vi "Create Test Method Dialog.vi"(8 "Error In":errorcluster, 11 "Class Ref":refnum<vi>) -> (0 "Error Out":errorcluster, 3 "Cancelled?":bool)   [LabVIEW 2013, in "Scripter.lvlib"]
uses:
  Scripter.lvlib
  _td Dialog Data.ctl
panel:
  in  "_btn Cancel":bool
  in  "_btn OK":bool
  in  "Templates List":u16(ring) items=["test template standart"]
  in  "Use Template?":bool
  out "Log Message":string
  in  "New Test Method Name":string
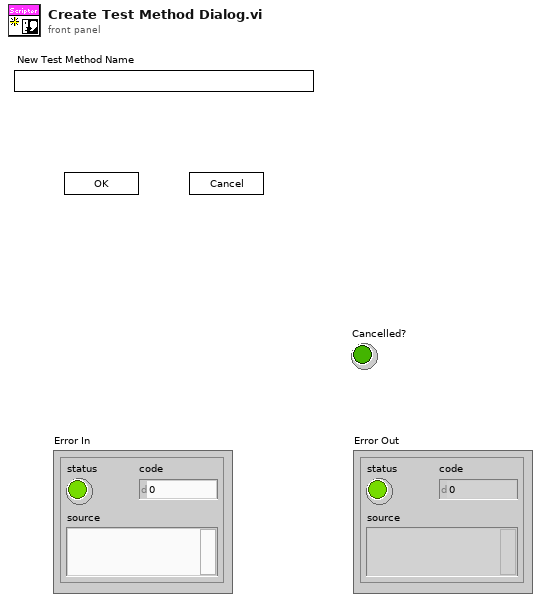
[diagram p1: front panel]
types:
  T1 = enum32{"Invalid", "Standard", "Closed", "Hidden", "Minimized", "Maximized"}
  T2 = enum32{"invalid app kind", "Development System", "Run Time System", "Student Edition", "Embedded LabVIEW", "Evaluation", "Custom"}
  T3 = typedef "Scripter.lvlib/_td Dialog Data.ctl" = cluster{"Core":cluster{"Current VI Reference":refnum<vi>, "Close Panel on Exit?":bool}, "Class Ref":refnum<vi>, "Class Folder Path":path, "Method Name":string, "Methods List":string[], "Templates Folder Path":path, "Template VIs":path[], "Template VIs List":string[], "Use Template?":bool, "Cancelled":bool, "Log Msg":string, "Validation Status":bool, "New Method Path":path, "Class Path":path, "VI Ref":refnum<vi>, "Default Template":path, "Method Idx":i32}
  T4 = enum8{"Enabled", "Disabled", "Disabled and Grayed Out"}
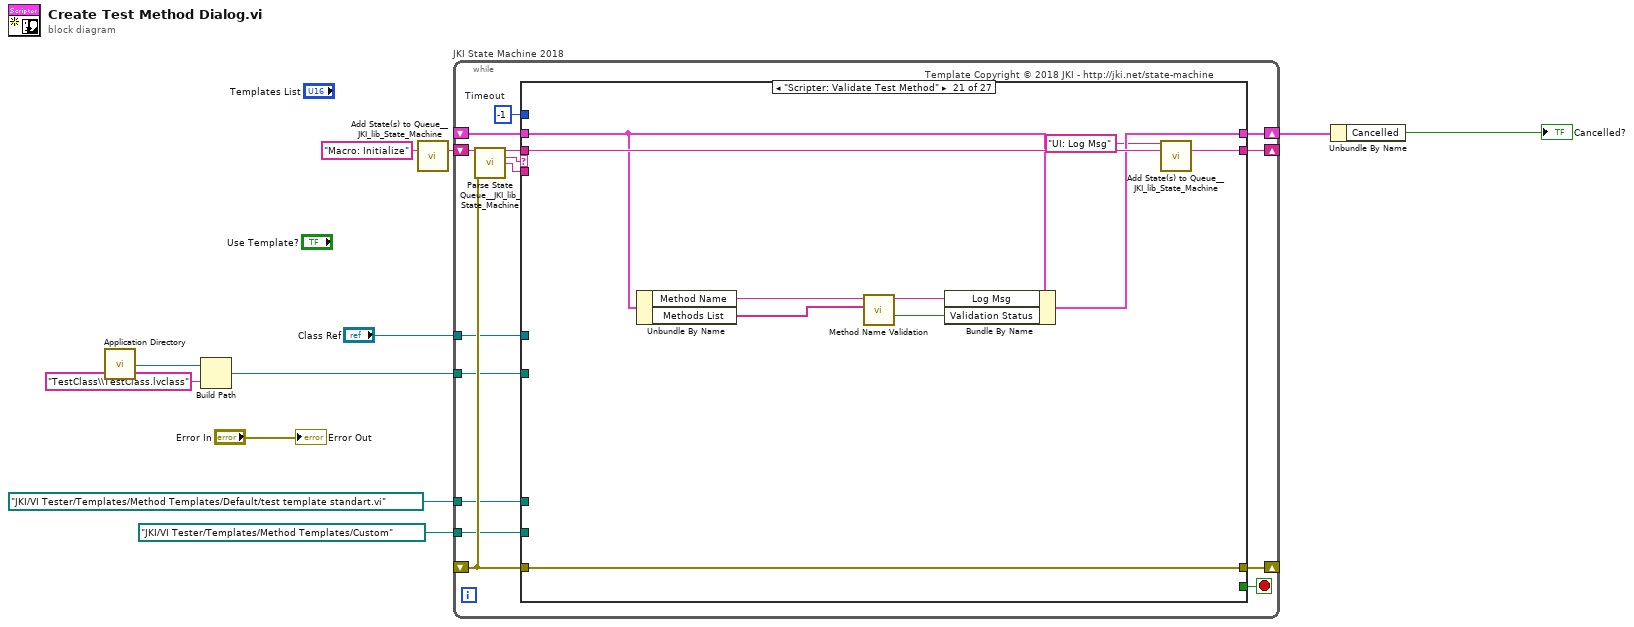
[diagram p0: block diagram]
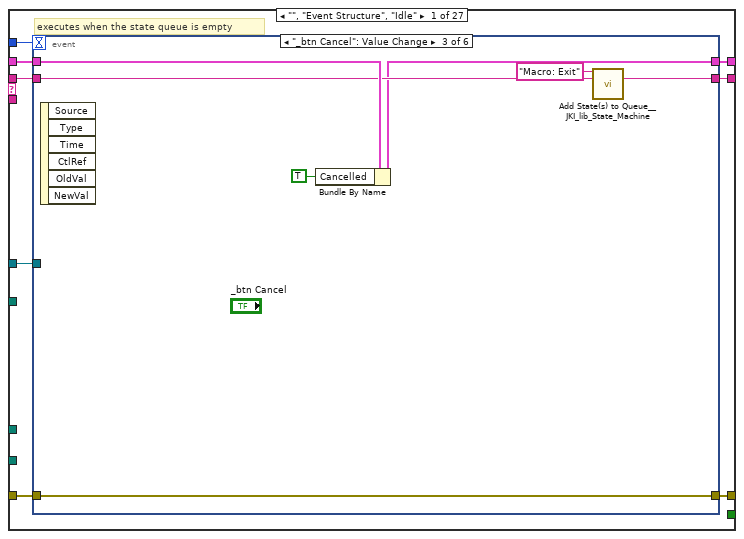
[diagram p2: hidden frame]
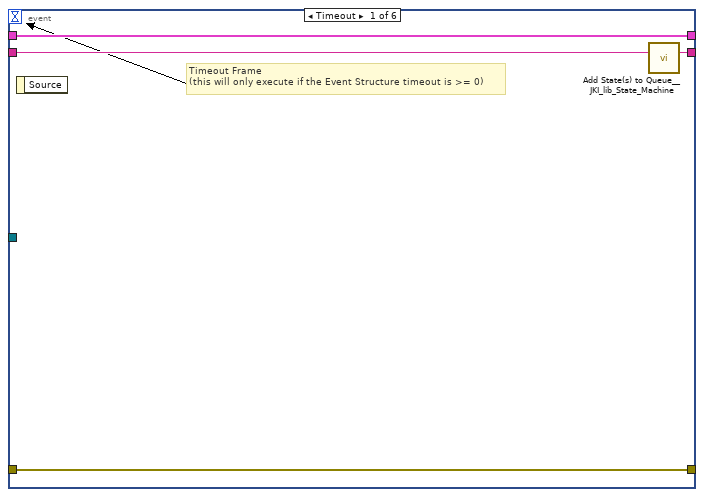
[diagram p3: hidden frame]
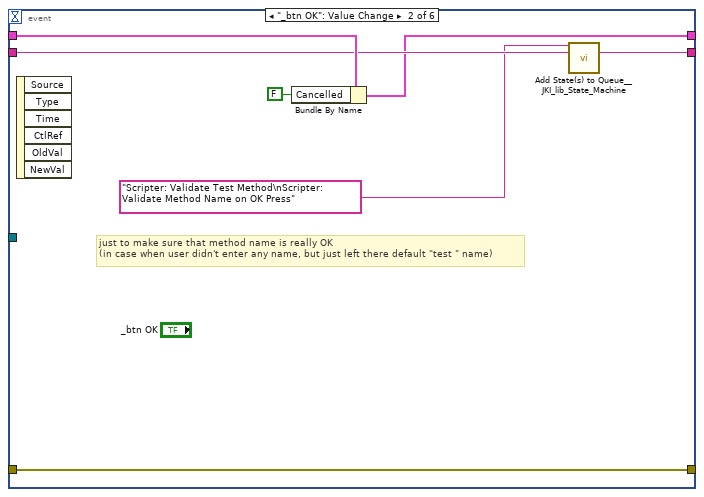
[diagram p4: hidden frame]
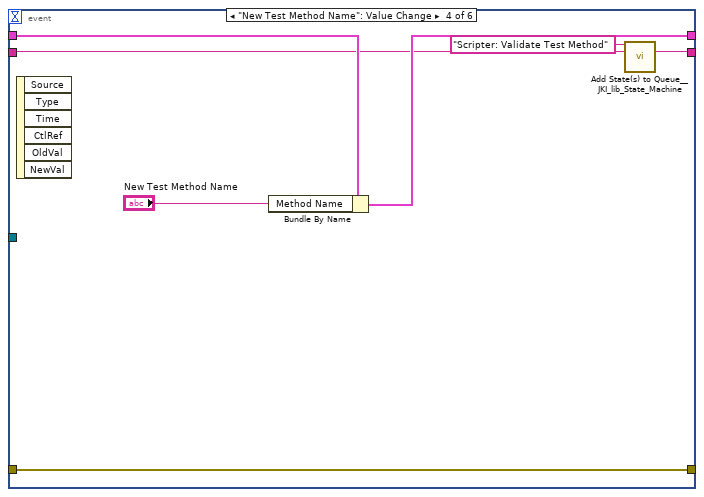
[diagram p5: hidden frame]
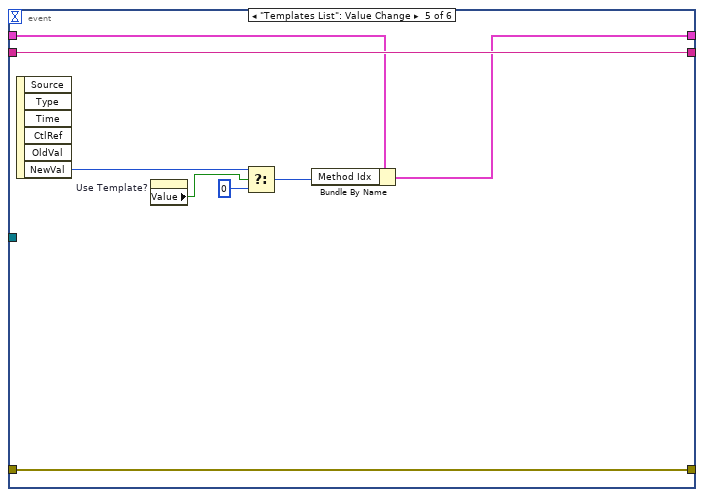
[diagram p6: hidden frame]
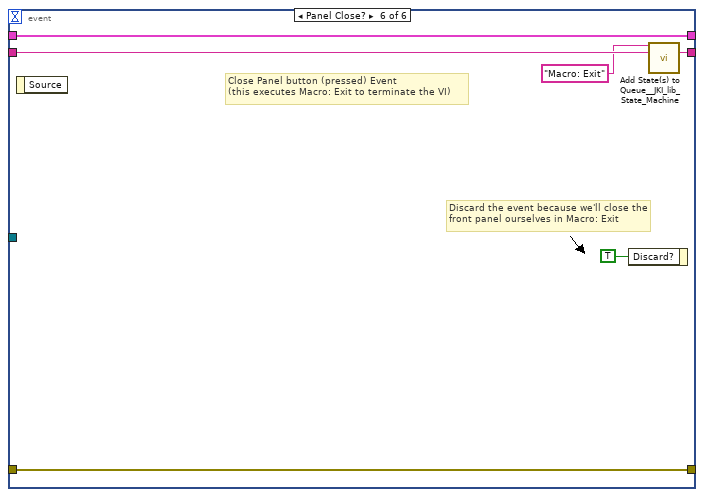
[diagram p7: hidden frame]
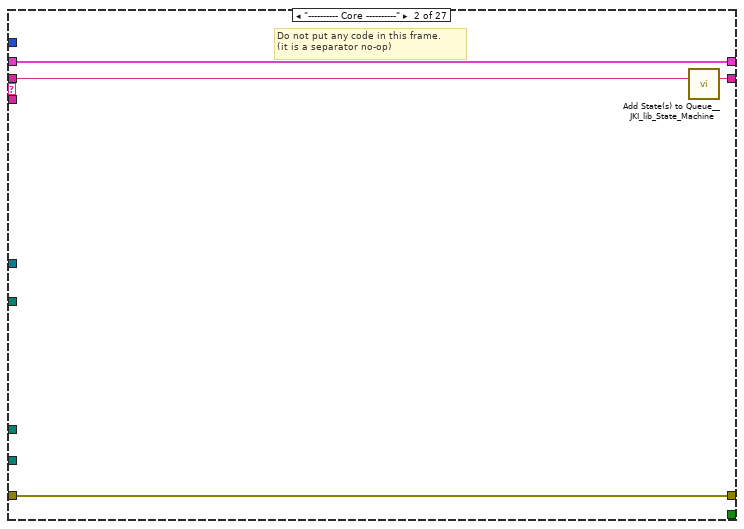
[diagram p8: hidden frame]
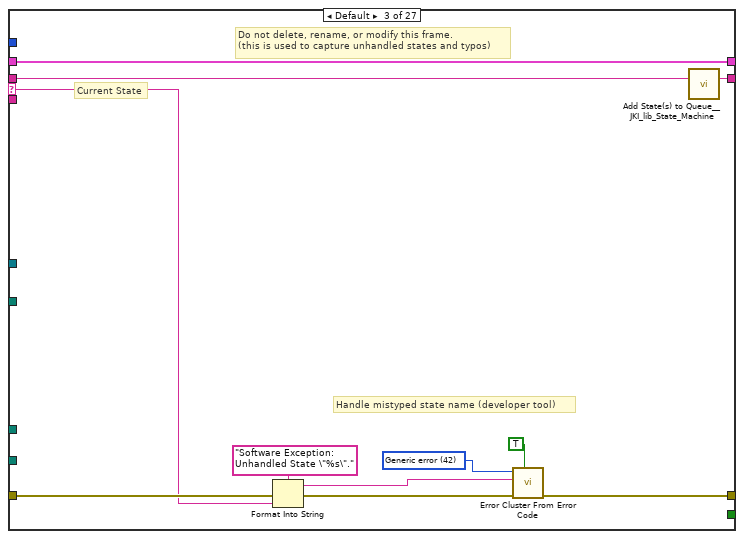
[diagram p9: hidden frame]
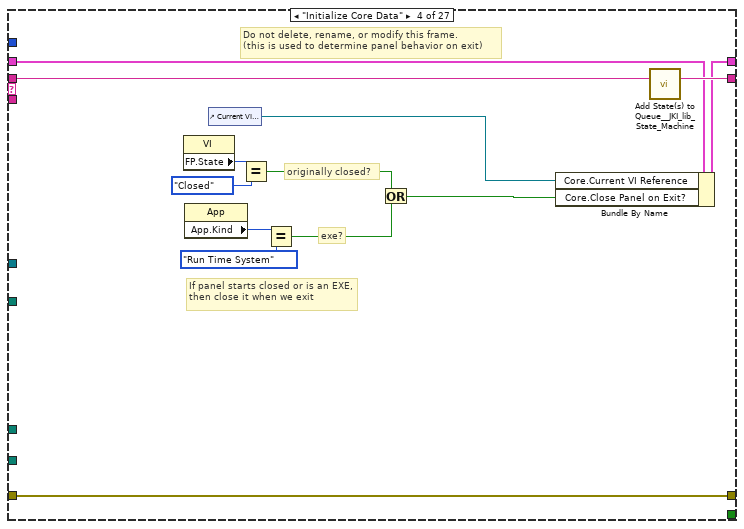
[diagram p10: hidden frame]
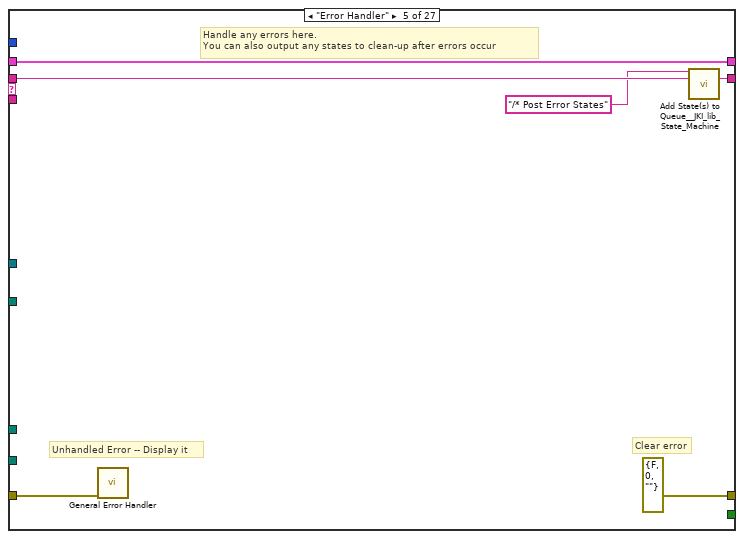
[diagram p11: hidden frame]
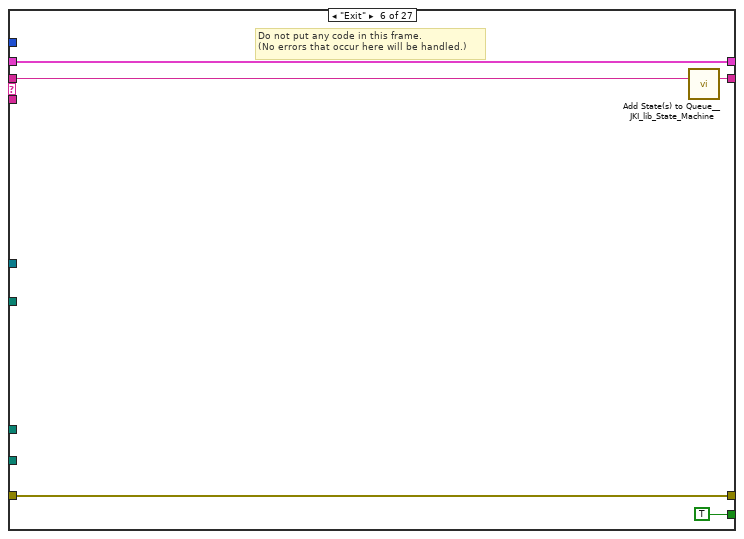
[diagram p12: hidden frame]
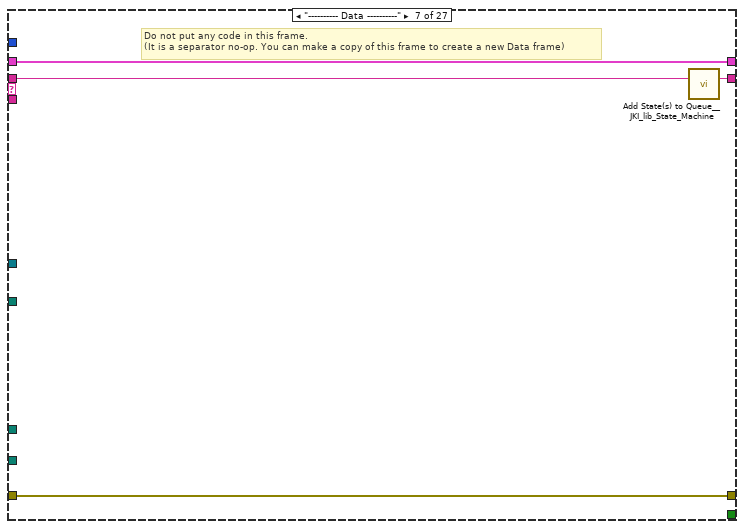
[diagram p13: hidden frame]
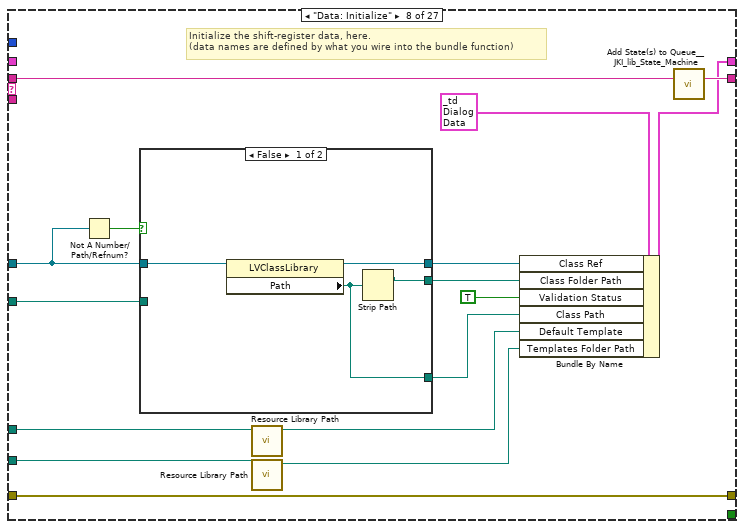
[diagram p14: hidden frame]
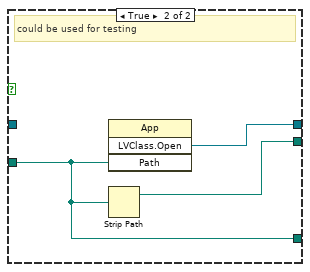
[diagram p15: hidden frame]
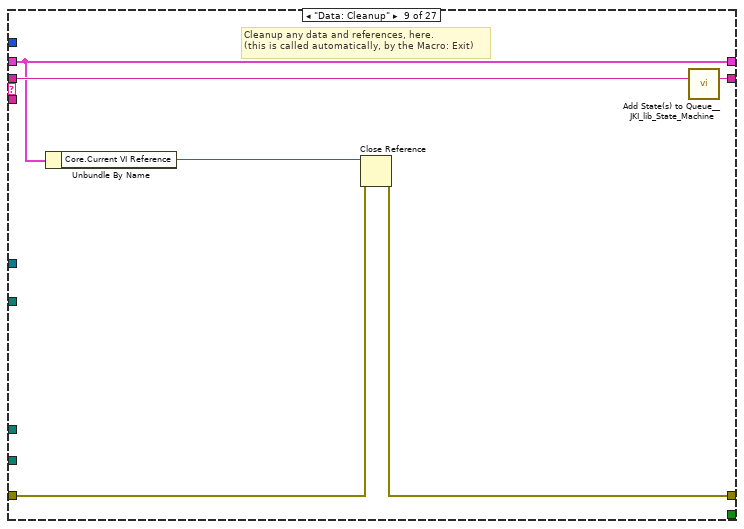
[diagram p16: hidden frame]
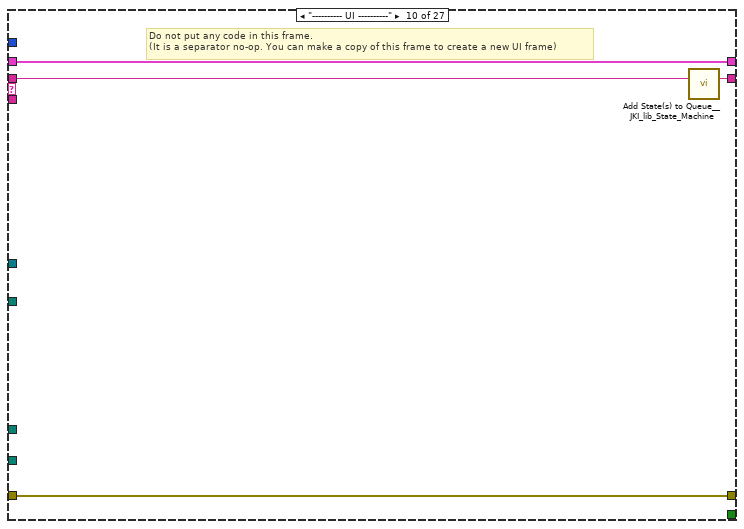
[diagram p17: hidden frame]
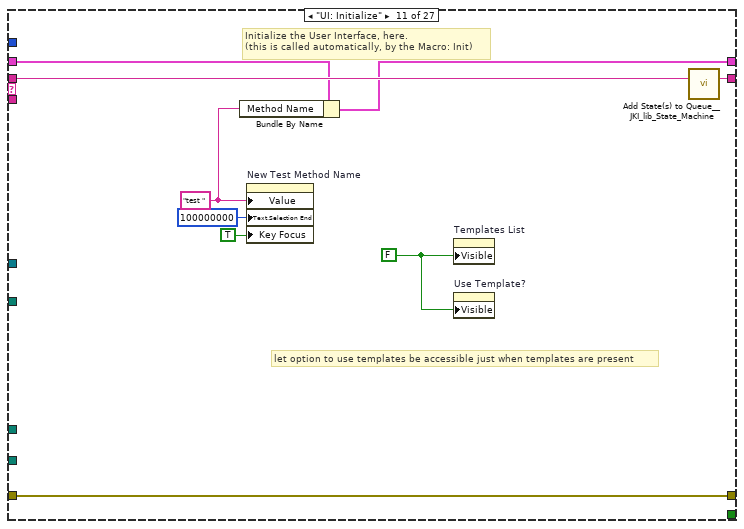
[diagram p18: hidden frame]
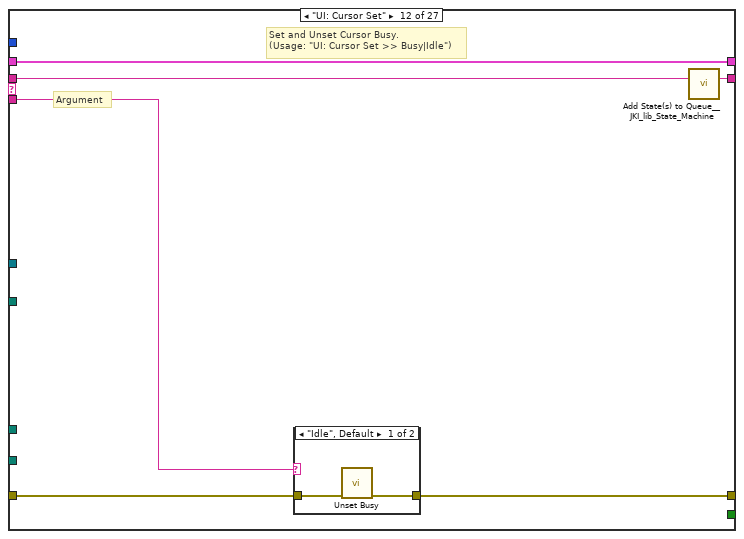
[diagram p19: hidden frame]
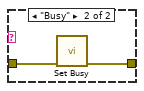
[diagram p20: hidden frame]
diagram:
  n1 = call <vilib>:"Application Directory.vi"() -> ("Application Directory"=w6:path)
  n2 = Build Path(base path=w6, name or relative path="TestClass\\TestClass.lvclass") -> (appended path=w4:path)
  n3 = call <vilib>:"Add State(s) to Queue__JKI_lib_State_Machine.vi"("State(s) in (\"\")"="Macro: Initialize") -> ("States Out"=w11:string)  [unwired: 14 in]
  n4 = while "JKI State Machine 2018" {
    shift-right: [w19] -> w8
    shift-left: _ -> [w18]
    shift-right: [w22] -> _
    shift-left: _ -> [w16]
    shift-right: [w21] -> _
    shift-left: w11 -> [w23]
    tunnel: "Class Ref" -> [w15]
    tunnel: w4 -> [w14]
    tunnel: path "JKI/VI Tester/Templates/Method Templates/Default/test template standart.vi" ("Relative Path") -> [w13]
    tunnel: path "JKI/VI Tester/Templates/Method Templates/Custom" ("Relative Path") -> [w12]
    stop <- w20 stop-if-true
    w17 = -1  # Timeout
    # "Template Copyright © 2018 JKI - http://jki.net/state-machine"
    n5 = call <vilib>:"Parse State Queue__JKI_lib_State_Machine.vi"("State Queue"=w23, "Error In (no error)"=w16) -> ("Remaining States"=w25:string, "Current State"=w26:string, "Arguments"=w24:string)  [unwired: 11 in]
    n6 = case shown="\"Scripter: Validate Test Method\"" w26 {
      selector: w26 -> [_ _ w78 _ _ _ _ _ _ _ _ _ _ _ _ _ _ _ _ _ _ _ _ _ _ _ _]
      tunnel: w25 -> [w34 w77 w82 w101 w107 w112 w116 w132 w145 w149 w158 w164 w175 w249 w256 w262 w267 w272 w282 w286 w296 w304 w314 w330 w340 w352 w363]
      tunnel: w24 -> [_ _ _ _ _ _ _ _ _ _ _ w159 w169 _ _ _ _ _ _ _ _ _ _ _ _ _ _]
      tunnel: w18 -> [w32 w74 w80 w94 w104 w110 w113 _ w140 w146 w156 w162 w171 w246 w253 w259 w264 w269 w279 w283 w293 w301 w311 w324 w337 w350 w361]
      tunnel: [w31 w75 w84 w98 errorcluster {"status"=FALSE, "code"=0, "source"=""} ("error out") w109 w114 w130 w141 w147 w155 w160 w172 w247 w254 w260 w265 w270 w280 w284 w294 w302 w312 w328 w338 w344 w357] -> w22
      tunnel: w16 -> [w30 w75 w83 w98 w103 w109 w114 w130 w142 w147 w155 w161 w173 w247 w254 w260 w265 w270 w280 w284 w294 w302 w312 w328 w338 w345 w358]
      tunnel: [w33 w76 w81 w100 w106 w111 w115 w131 w144 w148 w157 w163 w174 w248 w255 w261 w266 w271 w281 w285 w295 w303 w313 w329 w339 w351 w362] -> w21
      tunnel: [_ _ _ _ _ TRUE _ _ _ _ _ _ _ _ _ _ _ _ _ _ _ _ _ _ _ _ _] -> w20
      tunnel: [w29 w74 w80 w99 w104 w110 w113 w128 w140 w146 w151 w162 w171 w246 w253 w259 w264 w269 w279 w283 w292 w301 w306 w327 w332 w343 w361] -> w19
      tunnel: w17 -> [w28 _ _ _ _ _ _ _ _ _ _ _ _ _ _ _ _ _ _ _ _ _ _ _ _ _ _]
      tunnel: w15 -> [w27 _ _ _ _ _ _ w126 _ _ _ _ _ _ _ _ _ _ _ _ _ _ _ _ _ _ _]
      tunnel: w14 -> [_ _ _ _ _ _ _ w124 _ _ _ _ _ _ _ _ _ _ _ _ _ _ _ _ _ _ _]
      tunnel: w13 -> [_ _ _ _ _ _ _ w119 _ _ _ _ _ _ _ _ _ _ _ _ _ _ _ _ _ _ _]
      tunnel: w12 -> [_ _ _ _ _ _ _ w118 _ _ _ _ _ _ _ _ _ _ _ _ _ _ _ _ _ _ _]
      frame "", "Event Structure", "Idle" {
        # "executes when the state queue is empty"
        n7 = event shown="[2] \"_btn Cancel\": Value Change" {
          selector: _ -> [_ _ _ _ _ _]
          dyn-events: _ -> [_ _ _ _ _ _]
          timeout: w28 -> [_ _ _ _ _ _]
          tunnel: w34 -> [w38 w42 w49 w54 w67 w73]
          tunnel: [w37 w43 w50 w55 w67 w72] -> w33
          tunnel: w32 -> [w35 w44 w51 w58 w65 w70]
          tunnel: [w36 w45 w52 w59 w66 w71] -> w31
          tunnel: w30 -> [w36 w45 w52 w59 w66 w71]
          tunnel: [w35 w40 w47 w57 w64 w70] -> w29
          tunnel: w27 -> [_ _ _ _ _ _]
          event Timeout {
            # "Timeout Frame\n(this will only execute if the Event Structure timeout is >= 0)"
            n8 = event-data() -> ()  [unwired: 1 in, 1 out]
            n9 = call <vilib>:"Add State(s) to Queue__JKI_lib_State_Machine.vi"("State(s) in (\"\")"=w38) -> ("States Out"=w37:string)  [unwired: 14 in]
          }
          event "_btn OK": Value Change {
            # "just to make sure that method name is really OK\n(in case when user didn't enter any name, but just left there default \"test \" name)"
            n10 = event-data() -> ()  [unwired: 1 in, 6 out]
            n11 = Bundle By Name(cluster=w44, "Cancelled"=FALSE) -> (w40:T3)
            n12 = call <vilib>:"Add State(s) to Queue__JKI_lib_State_Machine.vi"("State(s) in Front (\"\")"="Scripter: Validate Test Method\nScripter: Validate Method Name on OK Press" ("State(s) in Front (\"\")"), "State(s) in (\"\")"=w42) -> ("States Out"=w43:string)  [unwired: 13 in]
          }
          event "_btn Cancel": Value Change {
            n13 = event-data() -> ()  [unwired: 1 in, 6 out]
            n14 = Bundle By Name(cluster=w51, "Cancelled"=TRUE) -> (w47:T3)
            n15 = call <vilib>:"Add State(s) to Queue__JKI_lib_State_Machine.vi"("State(s) in Front (\"\")"="Macro: Exit" ("State(s) in Front (\"\")"), "State(s) in (\"\")"=w49) -> ("States Out"=w50:string)  [unwired: 13 in]
          }
          event "New Test Method Name": Value Change {
            n16 = event-data() -> ()  [unwired: 1 in, 6 out]
            n17 = Bundle By Name(cluster=w58, "Method Name"="New Test Method Name") -> (w57:T3)
            n18 = call <vilib>:"Add State(s) to Queue__JKI_lib_State_Machine.vi"("State(s) in Front (\"\")"="Scripter: Validate Test Method" ("State(s) in Front (\"\")"), "State(s) in (\"\")"=w54) -> ("States Out"=w55:string)  [unwired: 13 in]
          }
          event "Templates List": Value Change {
            n19 = event-data() -> ("NewVal"=w62:u16)  [unwired: 1 in, 5 out]
            n20 = property on="Use Template?" class="Bool (strict)"() -> ("Value"=w63:bool)  [unwired: 2 in, 2 out]
            n21 = Select(t=w62, s=w63, f=u16 0) -> (s? t:f=w61:u16)
            n22 = Bundle By Name(cluster=w65, "Method Idx"=w61) -> (w64:T3)
          }
          event Panel Close? {
            # "Discard the event because we'll close the front panel ourselves in Macro: Exit"
            # "Close Panel button (pressed) Event\n(this executes Macro: Exit to terminate the VI)"
            n23 = event-data() -> ()  [unwired: 1 in, 1 out]
            n24 = event-data("Discard?"=TRUE) -> ()  [unwired: 1 in, 1 out]
            n25 = call <vilib>:"Add State(s) to Queue__JKI_lib_State_Machine.vi"("State(s) in Front (\"\")"="Macro: Exit", "State(s) in (\"\")"=w73) -> ("States Out"=w72:string)  [unwired: 13 in]
          }
        }
      }
      frame "---------- Core ----------" {
        # "Do not put any code in this frame.\n(it is a separator no-op)"
        n26 = call <vilib>:"Add State(s) to Queue__JKI_lib_State_Machine.vi"("State(s) in (\"\")"=w77) -> ("States Out"=w76:string)  [unwired: 14 in]
      }
      frame Default {
        w87 = 42 items=["No error", "Argument error", "Memory is full", "Out of zone", "End of file", "File already open", "Generic file I/O error", "File not found", "File permission error", "Disk is full", "Duplicate path", "Too many files open", "System feature not enabled", "Resource file not found", "Cannot add resource", "Resource not found", "Image not found", "Image memory error", "Pen does not exist", "Config type invalid", "Config token not found", "Config parse error", "Config memory error", "Bad external code format", "Bad external code offset", "External code not present", "Null window", "Destroy window error", "Null menu", "Print aborted", "Bad print record", "Print driver error", "Windows error during printing", "Memory error during printing", "Print dialog error", "Generic print error", "Invalid device refnum", "Device not found", "Device parameter error", "Device unit error", "Cannot open device", "Device call aborted", "Generic error", "Cancelled by user", "Object ID too low", "Object ID too high", "Object not in heap", "Unknown heap", "Unknown object (invalid DefProc)", "Unknown object (DefProc not in table)", "Message out of range", "Invalid (null) method", "Unknown message", "Manager call not supported", "Bad address", "Network operation in progress", "Network operation timed out", "Connection is busy", "Network attribute not supported", "Network error", "Address in use", "System out of memory", "Connection aborted", "Connection refused", "Not connected", "Already connected", "Connection closed", "Initialization error (interapplication manager)", "Bad occurrence", "Wait on unbound occurrence handler", "Occurrence queue overflow", "Datalog type conflict", "Unused", "Unrecognized type (interapplication manager)", "Memory corrupt", "Failed to make temporary DLL", "Old CIN version", "Drag socket not found", "Failed to load drop-object", "Failed to register OLE object", "Failed to release OLE object", "Format specifier type mismatch", "Unknown format specifier", "Too few format specifiers", "Too many format specifiers", "Scan failed", "Newer CIN version", "Error converting to variant", "Runtime menu error", "Password tampered", "Variant attribute not found", "Incompatible variant data type", "Event data is not available", "Event Store is not present", "Occurrence is not found", "Event Queue is not created", "Event info is not available", "Refnum passed is NULL", "Error retrieving Class GUID", "Error retrieving CoClass GUID", "Error retrieving TypeLib GUID.", "Bad built application magic bytes.", "Specific driver is different from the specific driver associated with the Logical Name.", "There is no session opened to the class driver.", "Max Error", "MAX - Error with config objects", "MAX - Error loading configuration", "MAX - Group not supported"]
        # "Current State"
        # "Do not delete, rename, or modify this frame.\n(this is used to capture unhandled states and typos)"
        # "Handle mistyped state name (developer tool)"
        n27 = Format Into String(format string="Software Exception: Unhandled State \"%s\"." ("message"), error in=w83, w78) -> (resulting string=w86:string, error out=w85:errorcluster)  [unwired: 1 in]
        n28 = call <vilib>:"Error Cluster From Error Code.vi"("show call chain? (False)"=TRUE, "error in (no error)"=w85, "error message (\"\")"=w86, "error code (0)"=w87) -> ("error out"=w84:errorcluster)  [unwired: 5 in]
        n29 = call <vilib>:"Add State(s) to Queue__JKI_lib_State_Machine.vi"("State(s) in (\"\")"=w82) -> ("States Out"=w81:string)  [unwired: 14 in]
      }
      frame "Initialize Core Data" {
        # "Do not delete, rename, or modify this frame.\n(this is used to determine panel behavior on exit)"
        # "originally closed?"
        # "exe?"
        # "If panel starts closed or is an EXE, then close it when we exit"
        n30 = property class="VI"() -> ("FP.State"=w91:T1)  [unwired: 2 in, 2 out]
        n31 = property class="App"() -> ("App.Kind"=w97:T2)  [unwired: 2 in, 2 out]
        n32 = control-ref of="Current VI Reference"() -> (w92:refnum<vi>)
        n33 = Equal?(x=w91, y=T1."Closed" ("Front Panel Window:State")) -> (x = y?=w89:bool)
        n34 = Equal?(x=w97, y=T2."Run Time System" ("Application:Kind")) -> (x = y?=w95:bool)
        n35 = Or(x=w89, y=w95) -> (x .or. y?=w93:bool)
        n36 = Bundle By Name(cluster=w94, "Core.Current VI Reference"=w92, "Core.Close Panel on Exit?"=w93) -> (w99:T3)
        n37 = call <vilib>:"Add State(s) to Queue__JKI_lib_State_Machine.vi"("State(s) in (\"\")"=w101) -> ("States Out"=w100:string)  [unwired: 14 in]
      }
      frame "Error Handler" {
        # "Unhandled Error -- Display it"
        # "Handle any errors here.\nYou can also output any states to clean-up after errors occur"
        # "Clear error"
        n38 = call <vilib>:"General Error Handler.vi"("error in (no error)"=w103) -> ()  [unwired: 10 in, 5 out]
        n39 = call <vilib>:"Add State(s) to Queue__JKI_lib_State_Machine.vi"("State(s) in Front (\"\")"="/* Post Error States", "State(s) in (\"\")"=w107) -> ("States Out"=w106:string)  [unwired: 13 in]
      }
      frame "Exit" {
        # "Do not put any code in this frame.\n(No errors that occur here will be handled.)"
        n40 = call <vilib>:"Add State(s) to Queue__JKI_lib_State_Machine.vi"("State(s) in (\"\")"=w112) -> ("States Out"=w111:string)  [unwired: 14 in]
      }
      frame "---------- Data ----------" {
        # "Do not put any code in this frame.\n(It is a separator no-op. You can make a copy of this frame to create a new Data frame)"
        n41 = call <vilib>:"Add State(s) to Queue__JKI_lib_State_Machine.vi"("State(s) in (\"\")"=w116) -> ("States Out"=w115:string)  [unwired: 14 in]
      }
      frame "Data: Initialize" {
        # "Initialize the shift-register data, here.\n(data names are defined by what you wire into the bundle function)"
        n42 = Not A Number/Path/Refnum?(number/path/refnum=w126) -> (NaN/Path/Refnum?=w127:bool)
        n43 = case shown="False" w127 {
          tunnel: w126 -> [w136 _]
          tunnel: [w135 w139] -> w125
          tunnel: w124 -> [_ w137]
          tunnel: [w134 w138] -> w123
          tunnel: [w133 w137] -> w121
          frame False {
            n44 = property class="LVClassLibrary"(reference=w136) -> (reference out=w135:refnum<vi>, "Path"=w133:path)  [unwired: 1 in, 1 out]
            n45 = Strip Path(path=w133) -> (stripped path=w134:path)  [unwired: 1 out]
          }
          frame True {
            # "could be used for testing"
            n46 = invoke class="App" method="LVClass.Open"("Path"=w137) -> ("LVClass.Open"=w139:refnum<vi>)  [unwired: 3 in, 3 out]
            n47 = Strip Path(path=w137) -> (stripped path=w138:path)  [unwired: 1 out]
          }
        }
        n48 = call "Resource Library Path.vi"("Relative Path"=w119) -> ("Resource + Relative Path"=w120:path)  [unwired: 10 in]
        n49 = call "Resource Library Path.vi"("Relative Path"=w118) -> ("Resource + Relative Path"=w117:path)  [unwired: 10 in]
        n50 = Bundle By Name(cluster=T3 {"Core"={"Current VI Reference"=refnum, "Close Panel on Exit?"=FALSE}, "Class Ref"=refnum, "Class Folder Path"=path "", "Method Name"="", "Methods List"=[], "Templates Folder Path"=path "", "Template VIs"=[], "Template VIs List"=[], "Use Template?"=FALSE, "Cancelled"=FALSE, "Log Msg"="", "Validation Status"=FALSE, "New Method Path"=path "", "Class Path"=path "", "VI Ref"=refnum, "Default Template"=path "", "Method Idx"=0} ("Dialog Data"), "Class Ref"=w125, "Class Folder Path"=w123, "Validation Status"=TRUE, "Class Path"=w121, "Default Template"=w120, "Templates Folder Path"=w117) -> (w128:T3)
        n51 = call <vilib>:"Add State(s) to Queue__JKI_lib_State_Machine.vi"("State(s) in (\"\")"=w132) -> ("States Out"=w131:string)  [unwired: 14 in]
      }
      frame "Data: Cleanup" {
        # "Cleanup any data and references, here.\n(this is called automatically, by the Macro: Exit)"
        n52 = Unbundle By Name(w140) -> ("Core.Current VI Reference"=w143:refnum<vi>)
        n53 = Close Reference(reference=w143, error in (no error)=w142) -> (error out=w141:errorcluster)
        n54 = call <vilib>:"Add State(s) to Queue__JKI_lib_State_Machine.vi"("State(s) in (\"\")"=w145) -> ("States Out"=w144:string)  [unwired: 14 in]
      }
      frame "---------- UI ----------" {
        # "Do not put any code in this frame.\n(It is a separator no-op. You can make a copy of this frame to create a new UI frame)"
        n55 = call <vilib>:"Add State(s) to Queue__JKI_lib_State_Machine.vi"("State(s) in (\"\")"=w149) -> ("States Out"=w148:string)  [unwired: 14 in]
      }
      frame "UI: Initialize" {
        w150 = "test " ("New Test Method Name")
        w154 = FALSE ("Visible")
        # "let option to use templates be accessible just when templates are present"
        # "Initialize the User Interface, here.\n(this is called automatically, by the Macro: Init)"
        n56 = Bundle By Name(cluster=w156, "Method Name"=w150) -> (w151:T3)
        n57 = property on="New Test Method Name" class="Str"("Value"=w150, "Text.Selection End"=u32 100000000 ("Text.Selection:End"), "Key Focus"=TRUE) -> ()  [unwired: 2 in, 2 out]
        n58 = property on="Templates List" class="Ring (strict)"("Visible"=w154) -> ()  [unwired: 2 in, 2 out]
        n59 = property on="Use Template?" class="Bool (strict)"("Visible"=w154) -> ()  [unwired: 2 in, 2 out]
        n60 = call <vilib>:"Add State(s) to Queue__JKI_lib_State_Machine.vi"("State(s) in (\"\")"=w158) -> ("States Out"=w157:string)  [unwired: 14 in]
      }
      frame "UI: Cursor Set" {
        # "Argument"
        # "Set and Unset Cursor Busy.\n(Usage: \"UI: Cursor Set >> Busy|Idle\")"
        n61 = case shown="\"Idle\", Default" w159 {
          tunnel: w161 -> [w166 w168]
          tunnel: [w165 w167] -> w160
          frame "Idle", Default {
            n62 = call <vilib>:"Unset Busy.vi"("error in (no error)"=w166) -> ("error out"=w165:errorcluster)  [unwired: 10 in]
          }
          frame "Busy" {
            n63 = call <vilib>:"Set Busy.vi"("error in (no error)"=w168) -> ("error out"=w167:errorcluster)  [unwired: 9 in, 1 out]
          }
        }
        n64 = call <vilib>:"Add State(s) to Queue__JKI_lib_State_Machine.vi"("State(s) in (\"\")"=w164) -> ("States Out"=w163:string)  [unwired: 14 in]
      }
      frame "UI: Front Panel State" {
        # "Argument"
        # "Set Front Panel Open or Closed\n(Usage: \"UI: Front Panel State >> Open|Close\")"
        n65 = Unbundle By Name(w171) -> ("Core.Current VI Reference"=w170:refnum<vi>)
        n66 = case shown="\"Open\", \"Standard\", Default" w169 {
          tunnel: w173 -> [w181 w196 w207 w220 w233]
          tunnel: [w183 w197 w209 w222 w235] -> w172
          tunnel: w170 -> [w182 w194 w208 w221 w234]
          frame "Open", "Standard", Default {
            w176 = T1."Standard" ("State")
            n67 = property class="VI"(reference=w182, error in=w181) -> (reference out=w179:refnum<vi>, error out=w180:errorcluster, "FP.State"=w178:T1)
            n68 = Not Equal?(x=w178, y=w176) -> (x != y?=w177:bool)
            n69 = case shown="True" w177 {
              tunnel: [w187 w189] -> w183
              tunnel: w180 -> [w186 w189]
              tunnel: w179 -> [w185 _]
              tunnel: w176 -> [w184 _]
              frame True {
                n70 = invoke class="VI" method="FP.Open"(reference=w185, error in=w186, "Activate"=TRUE, "State"=w184) -> (error out=w187:errorcluster)  [unwired: 1 in, 4 out]
              }
              frame False {
              }
            }
          }
          frame "Close", "Closed" {
            n71 = property class="VI"(reference=w194, error in=w196) -> (reference out=w193:refnum<vi>, error out=w195:errorcluster, "FP.State"=w191:T1)
            n72 = Not Equal?(x=w191, y=T1."Closed" ("Front Panel Window:State")) -> (x != y?=w190:bool)
            n73 = case shown="True" w190 {
              tunnel: [w198 w201] -> w197
              tunnel: w195 -> [w198 w200]
              tunnel: w193 -> [_ w199]
              frame False {
              }
              frame True {
                n74 = invoke class="VI" method="FP.Close"(reference=w199, error in=w200) -> (error out=w201:errorcluster)  [unwired: 1 in, 2 out]
              }
            }
          }
          frame "Hidden", "Hide" {
            w202 = T1."Hidden" ("State")
            n75 = property class="VI"(reference=w208, error in=w207) -> (reference out=w205:refnum<vi>, error out=w206:errorcluster, "FP.State"=w204:T1)
            n76 = Not Equal?(x=w204, y=w202) -> (x != y?=w203:bool)
            n77 = case shown="True" w203 {
              tunnel: [w213 w214] -> w209
              tunnel: w206 -> [w212 w214]
              tunnel: w205 -> [w211 _]
              tunnel: w202 -> [w210 _]
              frame True {
                n78 = invoke class="VI" method="FP.Open"(reference=w211, error in=w212, "State"=w210) -> (error out=w213:errorcluster)  [unwired: 2 in, 4 out]
              }
              frame False {
              }
            }
          }
          frame "Minimize", "Minimized" {
            w215 = T1."Minimized" ("State")
            n79 = property class="VI"(reference=w221, error in=w220) -> (reference out=w218:refnum<vi>, error out=w219:errorcluster, "FP.State"=w217:T1)
            n80 = Not Equal?(x=w217, y=w215) -> (x != y?=w216:bool)
            n81 = case shown="True" w216 {
              tunnel: [w226 w227] -> w222
              tunnel: w219 -> [w225 w227]
              tunnel: w218 -> [w224 _]
              tunnel: w215 -> [w223 _]
              frame True {
                n82 = invoke class="VI" method="FP.Open"(reference=w224, error in=w225, "State"=w223) -> (error out=w226:errorcluster)  [unwired: 2 in, 4 out]
              }
              frame False {
              }
            }
          }
          frame "Maximize", "Maximized" {
            w228 = T1."Maximized" ("State")
            n83 = property class="VI"(reference=w234, error in=w233) -> (reference out=w231:refnum<vi>, error out=w232:errorcluster, "FP.State"=w230:T1)
            n84 = Not Equal?(x=w230, y=w228) -> (x != y?=w229:bool)
            n85 = case shown="True" w229 {
              tunnel: [w239 w240] -> w235
              tunnel: w232 -> [w238 w240]
              tunnel: w231 -> [w237 _]
              tunnel: w228 -> [w236 _]
              frame True {
                n86 = invoke class="VI" method="FP.Open"(reference=w237, error in=w238, "State"=w236) -> (error out=w239:errorcluster)  [unwired: 2 in, 4 out]
              }
              frame False {
              }
            }
          }
        }
        n87 = call <vilib>:"Add State(s) to Queue__JKI_lib_State_Machine.vi"("State(s) in (\"\")"=w175) -> ("States Out"=w174:string)  [unwired: 14 in]
      }
      frame "UI: Log Msg" {
        n88 = Unbundle By Name(w246) -> ("Log Msg"=→"Log Message":string, "Validation Status"=w244:bool)
        n89 = Select(t=T4."Enabled" ("Disabled"), s=w244, f=T4."Disabled and Grayed Out" ("Disabled")) -> (s? t:f=w243:T4)
        n90 = property on="_btn OK" class="Bool"("DisabledEnum"=w243) -> ()  [unwired: 2 in, 2 out]
        n91 = call <vilib>:"Add State(s) to Queue__JKI_lib_State_Machine.vi"("State(s) in (\"\")"=w249) -> ("States Out"=w248:string)  [unwired: 14 in]
      }
      frame "UI: Display Templates List" {
        n92 = Unbundle By Name(w253) -> ("Template VIs"=w251:path[])
        n93 = for {
          tunnel: w251 -> [w258] mode=indexing
          tunnel: [w257] -> w250 mode=indexing
          n94 = call <vilib>:"Get File Extension.vi"("file"=w258) -> ("filename without extension"=w257:string)  [unwired: 7 in, 3 out]
        }
        n95 = property on="Templates List" class="Ring (strict)"("Strings []"=w250, "Value"=0) -> ()  [unwired: 2 in, 2 out]
        n96 = call <vilib>:"Add State(s) to Queue__JKI_lib_State_Machine.vi"("State(s) in (\"\")"=w256) -> ("States Out"=w255:string)  [unwired: 14 in]
      }
      frame "---------- Macro ----------" {
        # "Do not put any code in this frame.\n(It is a separator no-op. You can make a copy of this frame to create a new Macro frame)"
        n97 = call <vilib>:"Add State(s) to Queue__JKI_lib_State_Machine.vi"("State(s) in (\"\")"=w262) -> ("States Out"=w261:string)  [unwired: 14 in]
      }
      frame "Macro: Initialize" {
        w263 = "Data: Initialize\nInitialize Core Data\nUI: Initialize\nUI: Log Msg\nUI: Front Panel State >> Open\nScripter: Get Methods List\nScripter: Get Templates List"  # Data: Initialize Initialize Core Data UI: Initialize UI: Log Msg UI: Front Panel State >> Open Scripter: Get Methods List Scripter: Get Templates List
        # "Initialization Macro\n(This is called once, when the VI starts)"
        n98 = call <vilib>:"Add State(s) to Queue__JKI_lib_State_Machine.vi"("State(s) in Front (\"\")"=w263, "State(s) in (\"\")"=w267) -> ("States Out"=w266:string)  [unwired: 13 in]
      }
      frame "Macro: Add Test Method" {
        n99 = call <vilib>:"Add State(s) to Queue__JKI_lib_State_Machine.vi"("State(s) in Front (\"\")"="Scripter: Prepare Paths\nScripter: Generate VI\nScripter: Add VI to Class\nMacro: Exit" ("State(s) in Front (\"\")"), "State(s) in (\"\")"=w272) -> ("States Out"=w271:string)  [unwired: 13 in]
      }
      frame "Macro: Exit" {
        # "Exit Macro\n(This is called once, when the VI exits)"
        n100 = Unbundle By Name(w279) -> ("Core.Close Panel on Exit?"=w278:bool)
        n101 = Select(t="UI: Front Panel State >> Close", s=w278, f="") -> (s? t:f=w275:string)
        n102 = call <vilib>:"Add State(s) to Queue__JKI_lib_State_Machine.vi"("State(s) in (\"\")"=w275, "State(s) at Back (\"\")"="Data: Cleanup\nExit") -> ("States Out"=w273:string)  [unwired: 13 in]
        n103 = call <vilib>:"Add State(s) to Queue__JKI_lib_State_Machine.vi"("State(s) in Front (\"\")"=w273, "State(s) in (\"\")"=w282) -> ("States Out"=w281:string)  [unwired: 13 in]
      }
      frame "---------- Scripter ----------" {
        # "Template Separator\n(You can make a copy of, or modify, this frame)"
        n104 = call <vilib>:"Add State(s) to Queue__JKI_lib_State_Machine.vi"("State(s) in (\"\")"=w286) -> ("States Out"=w285:string)  [unwired: 14 in]
      }
      frame "Scripter: Validate Test Method" {
        n105 = Unbundle By Name(w293) -> ("Method Name"=w287:string, "Methods List"=w288:string[])
        n106 = call "Method Name Validation.vi"("Methods List in"=w288, "Method Name in"=w287) -> ("Validation Status out"=w289:bool, "Log Message out"=w291:string)  [unwired: 8 in]
        n107 = Bundle By Name(cluster=w293, "Log Msg"=w291, "Validation Status"=w289) -> (w292:T3)
        n108 = call <vilib>:"Add State(s) to Queue__JKI_lib_State_Machine.vi"("State(s) in Front (\"\")"="UI: Log Msg", "State(s) in (\"\")"=w296) -> ("States Out"=w295:string)  [unwired: 13 in]
      }
      frame "Scripter: Validate Method Name on OK Press" {
        # "Template Separator\n(You can make a copy of, or modify, this frame)"
        n109 = Unbundle By Name(w301) -> ("Validation Status"=w300:bool)
        n110 = Select(t="Macro: Add Test Method" ("State(s) in Front (\"\")"), s=w300, f="") -> (s? t:f=w297:string)
        n111 = call <vilib>:"Add State(s) to Queue__JKI_lib_State_Machine.vi"("State(s) in Front (\"\")"=w297, "State(s) in (\"\")"=w304) -> ("States Out"=w303:string)  [unwired: 13 in]
      }
      frame "Scripter: Get Methods List" {
        n112 = Unbundle By Name(w311) -> ("Class Ref"=w310:refnum<vi>)
        n113 = property class="LVClassLibrary"(reference=w310) -> ("Dynamic Member VIs"=w309:refnum<vi>[], "Static Member VIs"=w308:refnum<vi>[])  [unwired: 1 in, 2 out]
        n114 = Build Array (concatenate)(w309, w308) -> (w307:refnum<vi>[])
        n115 = for {
          tunnel: w307 -> [w317] mode=indexing
          tunnel: [w315] -> w305 mode=indexing
          n116 = property class="VI"(reference=w317) -> ("Path"=w316:path)  [unwired: 1 in, 2 out]
          n117 = call <vilib>:"Get File Extension.vi"("file"=w316) -> ("filename without extension"=w315:string)  [unwired: 7 in, 3 out]
        }
        n118 = Bundle By Name(cluster=w311, "Methods List"=w305) -> (w306:T3)
        n119 = call <vilib>:"Add State(s) to Queue__JKI_lib_State_Machine.vi"("State(s) in (\"\")"=w314) -> ("States Out"=w313:string)  [unwired: 14 in]
      }
      frame "Scripter: Get Templates List" {
        n120 = Unbundle By Name(w324) -> ("Default Template"=w321:path, "Templates Folder Path"=w323:path)
        n121 = call <vilib>:"Recursive File List.vi"("pattern"="*.vi", "Folder Path"=w323) -> ("All Files in Dir"=w320:path[])  [unwired: 5 in, 4 out]
        n122 = Build Array (concatenate)(w321, w320) -> (w319:path[])
        n123 = Empty Array?(array=w320) -> (empty?=w326:bool)
        n124 = Not(x=w326) -> (.not. x?=w325:bool)
        n125 = Bundle By Name(cluster=w324, "Template VIs"=w319) -> (w327:T3)
        n126 = property on="Templates List" class="Ring (strict)"("Visible"=w325) -> ()  [unwired: 2 in, 2 out]
        n127 = property on="Use Template?" class="Bool (strict)"("Visible"=w325) -> ()  [unwired: 2 in, 2 out]
        n128 = call <vilib>:"Add State(s) to Queue__JKI_lib_State_Machine.vi"("State(s) in Front (\"\")"="UI: Display Templates List" ("State(s) in Front (\"\")"), "State(s) in (\"\")"=w330) -> ("States Out"=w329:string)  [unwired: 13 in]
      }
      frame "Scripter: Prepare Paths" {
        n129 = Unbundle By Name(w337) -> ("Class Folder Path"=w333:path, "Method Name"=w336:string)
        n130 = Format Into String(format string="%s.vi", w336) -> (resulting string=w334:string)  [unwired: 2 in, 1 out]
        n131 = Build Path(base path=w333, name or relative path=w334) -> (appended path=w331:path)
        n132 = Bundle By Name(cluster=w337, "New Method Path"=w331) -> (w332:T3)
        n133 = call <vilib>:"Add State(s) to Queue__JKI_lib_State_Machine.vi"("State(s) in (\"\")"=w340) -> ("States Out"=w339:string)  [unwired: 14 in]
      }
      frame "Scripter: Generate VI" {
        # "Template Separator\n(You can make a copy of, or modify, this frame)"
        n134 = Unbundle By Name(w350) -> ("Template VIs"=w349:path[], "Method Idx"=w341:i32, "Class Path"=w347:path, "New Method Path"=w346:path)
        n135 = Index Array(array=w349, index=w341) -> (element=w348:path)
        n136 = call "Replace Class Inputs.vi"("Error In"=w345, "Target VI Path"=w346, "Target Class Path"=w347, "Template VI Path"=w348) -> ("Error Out"=w344:errorcluster, "VI Ref out"=w342:refnum<vi>)  [unwired: 6 in]
        n137 = Bundle By Name(cluster=w350, "VI Ref"=w342) -> (w343:T3)
        n138 = call <vilib>:"Add State(s) to Queue__JKI_lib_State_Machine.vi"("State(s) in (\"\")"=w352) -> ("States Out"=w351:string)  [unwired: 14 in]
      }
      frame "Scripter: Add VI to Class" {
        # "Template Separator\n(You can make a copy of, or modify, this frame)"
        n139 = Unbundle By Name(w361) -> ("Class Ref"=w353:refnum<vi>, "Class Ref"=w360:refnum<vi>, "New Method Path"=w359:path, "VI Ref"=w356:refnum<vi>)
        n140 = call "Add VI to class library.vi"("Error In"=w358, "VI Ref"=w356, "New method path"=w359, "Class Ref"=w360) -> ("Error Out"=w355:errorcluster)  [unwired: 7 in]
        n141 = call "Save Class Library.vi"("Error In"=w355, "Library Ref in"=w353) -> ("Error Out"=w354:errorcluster)  [unwired: 9 in]
        n142 = Close Reference(reference=w356, error in (no error)=w354) -> (error out=w357:errorcluster)
        n143 = call <vilib>:"Add State(s) to Queue__JKI_lib_State_Machine.vi"("State(s) in (\"\")"=w363) -> ("States Out"=w362:string)  [unwired: 14 in]
      }
    }
  }
  n144 = Unbundle By Name(w8) -> ("Cancelled"=→"Cancelled?":bool)
  "Error Out" <- "Error In"
